vi "TC_J_VtoC.vi"(11 "Thermocouple Voltage":dbl caption="热电偶电压" format="%0.6f") -> (3 "T(c)":dbl format="%#_16f")   [LabVIEW 2012]
doc: "功能：\n\nE型热电偶电压转换为摄氏度。\n\ncsxcs_366创建。"
uses:
  <vilib>/Analysis/polynomials.llb/Scalar Polynomial Evaluation (DBL).vi
  <vilib>/Analysis/NI_AALPro.lvlib
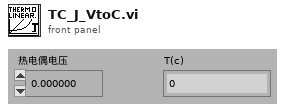
[diagram p1: front panel]
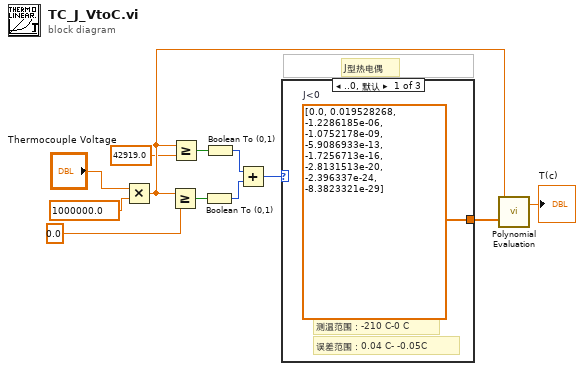
[diagram p0: block diagram]
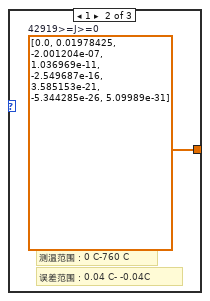
[diagram p2: hidden frame]
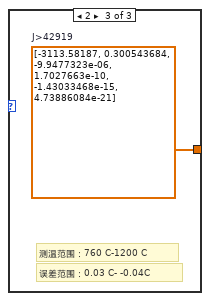
[diagram p3: hidden frame]
diagram:
  # "J型热电偶"
  n1 = Multiply(x="Thermocouple Voltage", y=1000000.0) -> (x*y=w8:dbl)
  n2 = Greater Or Equal?(x=w8, y=0.0) -> (x >= y?=w5:bool)
  n3 = Greater Or Equal?(x=w8, y=42919.0) -> (x >= y?=w6:bool)
  n4 = Boolean To (0,1)(Boolean=w5) -> (0, 1=w4:i16)
  n5 = Boolean To (0,1)(Boolean=w6) -> (0, 1=w3:i16)
  n6 = Add(x=w3, y=w4) -> (x+y=w2:i16)
  n7 = case shown="..0, 默认" w2 {
    tunnel: [w13 w14 w15] -> w1
    frame ..0, Default {
      w13 = dbl[] [0.0, 0.019528268, -1.2286185e-06, -1.0752178e-09, -5.9086933e-13, -1.7256713e-16, -2.8131513e-20, -2.396337e-24, -8.3823321e-29]  # J<0
      # "误差范围：0.04 C- -0.05C"
      # "测温范围：-210 C-0 C"
    }
    frame 1 {
      w14 = dbl[] [0.0, 0.01978425, -2.001204e-07, 1.036969e-11, -2.549687e-16, 3.585153e-21, -5.344285e-26, 5.09989e-31]  # 42919>=J>=0
      # "误差范围：0.04 C- -0.04C"
      # "测温范围：0 C-760 C"
    }
    frame 2 {
      w15 = dbl[] [-3113.58187, 0.300543684, -9.9477323e-06, 1.7027663e-10, -1.43033468e-15, 4.73886084e-21]  # J>42919
      # "误差范围：0.03 C- -0.04C"
      # "测温范围：760 C-1200 C"
    }
  }
  n8 = call-poly <vilib>:"Polynomial Evaluation.vi"("P(x)"=w1, "a"=w8) -> ("P(a)"=→"T(c)":dbl)  [unwired: 1 out]
